vi "SetAngle90.vi"(11 "Gear Manipulator.lvclass":refnum<class "Gear Manipulator.lvclass">) -> (3 "Gear Manipulator.lvclass":refnum<class "Gear Manipulator.lvclass">)   [LabVIEW 2016, in "Gear Manipulator.lvclass"]
uses:
  Gear Manipulator.lvclass
  Gear Manipulator.lvclass/Gear Manipulator.ctl
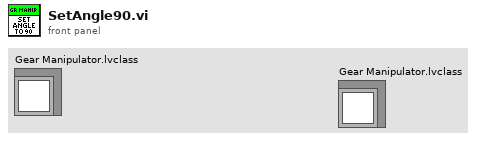
[diagram p1: front panel]
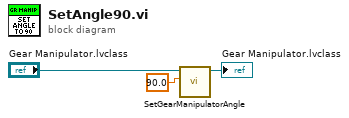
[diagram p0: block diagram]
diagram:
  n1 = call "SetGearManipulatorAngle.vi"("Gear Manipulator Angle"=90.0, "Gear Manipulator in"="Gear Manipulator.lvclass") -> ("Gear Manipulator out"=→"Gear Manipulator.lvclass":refnum<class "Gear Manipulator.lvclass">)  [unwired: 9 in]
